vi "DriveGetModuleRef.vi"(11 "ModualNamePrefix":i32) -> (0 "SpinMot":T2, 1 "SpinStr":string, 2 "TravMot":T2, 3 "TravStr":string, 4 "EncStr":string, 6 "EncDevice":T1)   [LabVIEW 2020]
uses:
  <vilib>/Rock Robotics/SystemInterfaces/DIO/FPGA_DIOPWMChannel.ctl
  <vilib>/Rock Robotics/WPI/PWM/WPI_PWMDeadband.ctl
  <vilib>/Rock Robotics/WPI/MotorControl/WPI_MotorControlType.ctl
  <vilib>/Rock Robotics/SystemInterfaces/DIO/FPGA_DIOChannel.ctl
  <vilib>/Rock Robotics/WPI/MotorControl/WPI_MotorControlDeviceRef.ctl
  <vilib>/Rock Robotics/WPI/ThirdParty/Phoenix-LabVIEW/CANCoder/Controls/CTRE_Phoenix_CANcoder_DeviceRef.ctl
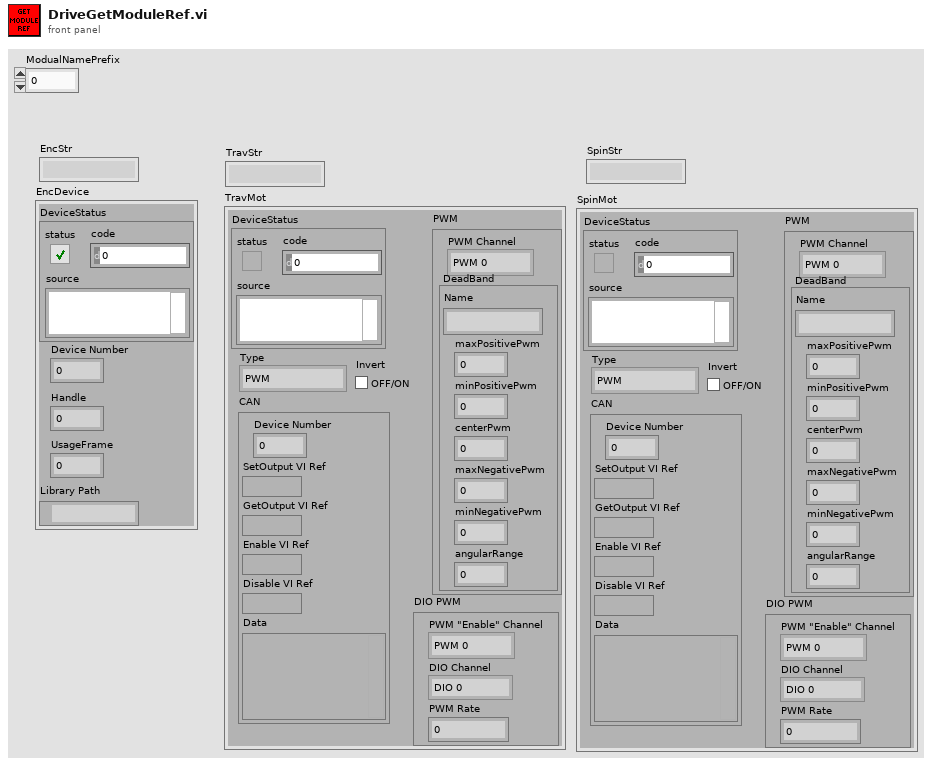
[diagram p1: front panel]
types:
  T1 = typedef "CTRE_Phoenix_CANcoder_DeviceRef.ctl" = cluster{"DeviceStatus":errorcluster, "Device Number":u8, "Handle":u64, "UsageFrame":u32, "Library Path":path}
  T2 = typedef "WPI_MotorControlDeviceRef.ctl" = cluster{"DeviceStatus":errorcluster, "Type":T3, "PWM":cluster{"PWM Channel":T4, "DeadBand":T5}, "CAN":cluster{"Device Number":u8, "SetOutput VI Ref":variant, "GetOutput VI Ref":variant, "Enable VI Ref":variant, "Disable VI Ref":variant, "Data":variant}, "Invert":bool, "DIO PWM":cluster{"PWM \"Enable\" Channel":T4, "DIOChannel":T6, "PWM Rate":dbl}}
  T3 = typedef "WPI_MotorControlType.ctl" = enum16{"PWM", "CAN", "DIO PWM"}
  T4 = typedef "FPGA_DIOPWMChannel.ctl" = enum8{"PWM 0", "PWM 1", "PWM 2", "PWM 3", "PWM 4", "PWM 5", "PWM 6", "PWM 7", "PWM 8", "PWM 9", "PWM MXP 0", "PWM MXP 1", "PWM MXP 2", "PWM MXP 3", "PWM MXP 4", "PWM MXP 5", "PWM MXP 6", "PWM MXP 7", "PWM MXP 8", "PWM MXP 9", "Invalid"}
  T5 = typedef "WPI_PWMDeadband.ctl" = cluster{"Name":string, "maxPositivePwm":i32, "minPositivePwm":i32, "centerPwm":i32, "maxNegativePwm":i32, "minNegativePwm":i32, "angularRange":u16}
  T6 = typedef "FPGA_DIOChannel.ctl" = enum8{"DIO 0", "DIO 1", "DIO 2", "DIO 3", "DIO 4", "DIO 5", "DIO 6", "DIO 7", "DIO 8", "DIO 9", "DIO MXP 0", "DIO MXP 1", "DIO MXP 2", "DIO MXP 3", "DIO MXP 4", "DIO MXP 5", "DIO MXP 6", "DIO MXP 7", "DIO MXP 8", "DIO MXP 9", "DIO MXP 10", "DIO MXP 11", "DIO MXP 12", "DIO MXP 13", "DIO MXP 14", "DIO MXP 15", "SPI Port CS1", "SPI Port CS2", "SPI Port CS3", "SPI Port MISO", "SPI Port MOSI", "Invalid"}
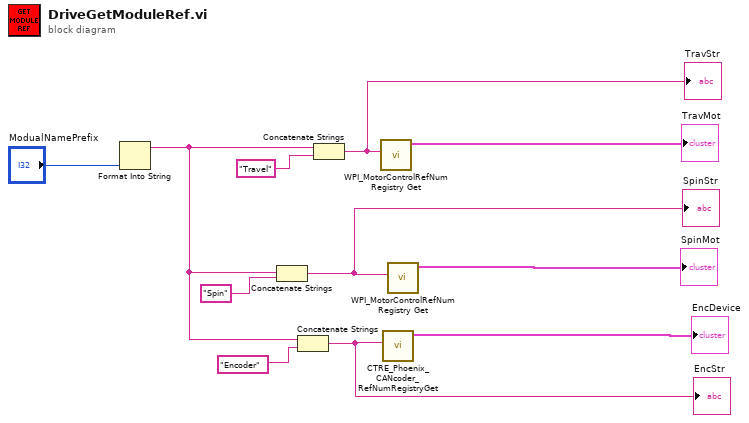
[diagram p0: block diagram]
diagram:
  n1 = Format Into String("ModualNamePrefix") -> (resulting string=w8:string)  [unwired: 3 in, 1 out]
  n2 = Concatenate Strings(w8, "Spin" ("refnum name")) -> (w10:string)
  "SpinStr" <- w10
  n3 = Concatenate Strings(w8, "Encoder" ("refnum name")) -> (w5:string)
  "EncStr" <- w5
  n4 = Concatenate Strings(w8, "Travel" ("refnum name")) -> (w11:string)
  "TravStr" <- w11
  n5 = call <vilib>:"WPI_MotorControlRefNum Registry Get.vi"("refnum name"=w11) -> ("MotorControlDevRef"=→"TravMot":T2)  [unwired: 9 in, 1 out]
  n6 = call <vilib>:"CTRE_Phoenix_CANcoder_RefNumRegistryGet.vi"("refnum name"=w5) -> ("CTRE_CANcoder_DeviceRef"=→"EncDevice":T1)  [unwired: 9 in, 1 out]
  n7 = call <vilib>:"WPI_MotorControlRefNum Registry Get.vi"("refnum name"=w10) -> ("MotorControlDevRef"=→"SpinMot":T2)  [unwired: 9 in, 1 out]
